vi "Query (Low Level).vi"(8 "error in":errorcluster, 9 "byte count":u32=4096 caption="byte count (4096)", 10 "Command":string, 11 "Mercury Reference In":T1) -> (0 "error out":errorcluster, 2 "Response":string, 3 "Comms out":refnum<visa-resource-name>)   [LabVIEW 2013, in "Mercury iXX.lvlib"]
uses:
  Mercury iXX.lvlib
  Public/Controls/Comms Transport Layer.ctl
  Public/Controls/Mercury Reference.ctl
  Controls/Query Dynamic Reference.ctl
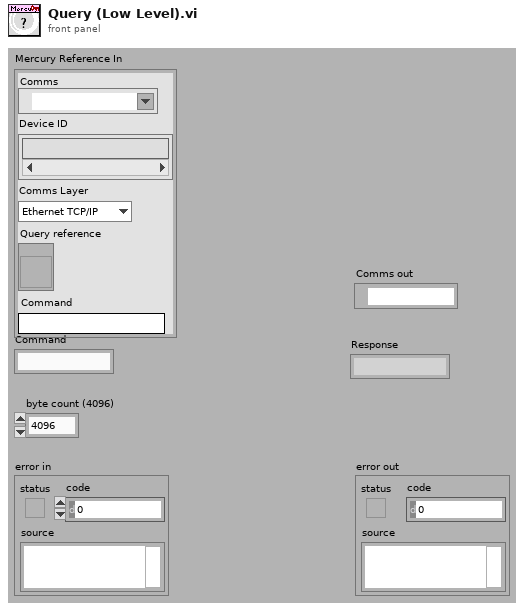
[diagram p1: front panel]
types:
  T1 = typedef "Mercury iXX.lvlib/Mercury Reference.ctl" = cluster{"Comms":refnum<visa-resource-name>, "Device ID":string[], "Comms Layer":T2, "Command":string, "Query reference":T3}
  T2 = typedef "Mercury iXX.lvlib/Comms Transport Layer.ctl" = enum16{"Ethernet TCP/IP", "USB", "ISOBus - RS-232", "GPIB"}
  T3 = typedef "Mercury iXX.lvlib/Query Dynamic Reference.ctl" = refnum<vi>
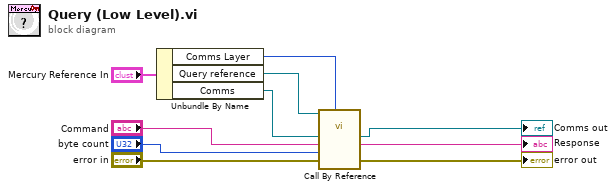
[diagram p0: block diagram]
diagram:
  n1 = Unbundle By Name("Mercury Reference In") -> ("Comms Layer"=w1:T2, "Query reference"=w2:T3, "Comms"=w3:refnum<visa-resource-name>)
  n2 = call-by-ref "?"(reference=w2, "Comms Layer"=w1, "error in"="error in", "byte count"="byte count", "Command"="Command", "Comms"=w3) -> ("error out"=→"error out":errorcluster, "Response"=→"Response":string, "Comms out"=→"Comms out":refnum<visa-resource-name>)  [unwired: 4 in, 3 out]
